vi "Generic - DI1.vi"(0 "VISA session":refnum<visa-resource-name>="MW100", 2 "Semiphore":T2, 5 "Channel_Enum":T1=1 items=["4-20_OUT", "Pres_HI1", "Pres_HI2", "Pres_LOW", "Pres_PIN", "HEATER_TOP", "HEATER_BOT", "T_Shell", "FLOWMETER", "WATT_SENSE", "WH_TICK", "Tc_1", "Tc_2", "Tc_3", "Tc_4", "Tc_5", "Tc_6", "Tc_down", "T_Shell_2", "T_Shell_3", "T_Shell_4", "RTD_IN", "RTD_OUT", "RTD_AMB", "INTF_TEMPFLO", "INTF_READY", "INTF_START", "INTF_STOP", "DRM_LOW", "DRM_HIGH", "PWR_MAIN", "VLV_DUMP", "VLV_OUT", "VLV_IN", "WATT_HOURS", "FLOW(SAMPLE)", "GALLONS", "FLOW(GPM)"], 11 "Error In":errorcluster) -> (4 "dup VISA session":refnum<visa-resource-name>, 6 "Value":bool, 15 "error out":errorcluster)   [LabVIEW 2009]
uses:
  ChannelSettings.ctl
panel:
  out "number":dbl
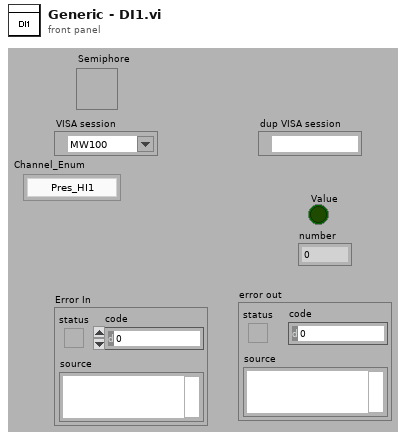
[diagram p1: front panel]
types:
  T1 = typedef "ChannelSettings.ctl" = u32
  T2 = typedef "Semaphore RefNum" = refnum<k1>
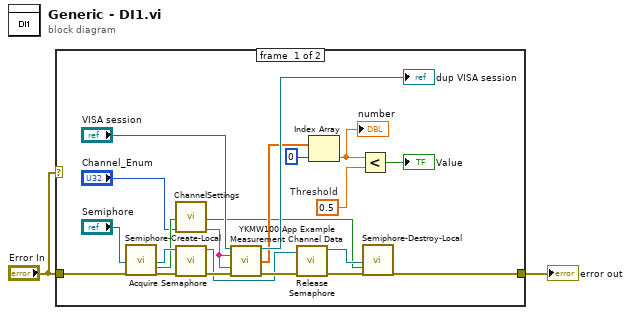
[diagram p0: block diagram]
diagram:
  n1 = case shown="Error" "Error In" {
    tunnel: "Error In" -> [w14 w23]
    tunnel: [w12 w23] -> w2
    frame #0 {
      w17 = 0.5  # Threshold
      n2 = call "Semiphore-Create-Local.vi"("Semiphore"="Semiphore", "error in (no error)"=w14) -> ("semaphore"=w9:T2, "Local?"=w4:bool, "error out"=w11:errorcluster)  [unwired: 15 in]
      n3 = call "ChannelSettings.vi"("Channel_Enum"="Channel_Enum") -> ("Channel String"=w20:string)  [unwired: 10 in]
      n4 = call <vilib>:"Acquire Semaphore.vi"("error in (no error)"=w11, "semaphore"=w9) -> ("error out"=w10:errorcluster, "semaphore out"=w6:T2)  [unwired: 3 in, 1 out]
      n5 = call "YKMW100 App Example Measurement Channel Data.vi"("VISA session"="VISA session", "Start Channel (001)"=w20, "End Channel (001)"=w20, "error in (no error)"=w10) -> ("dup VISA session"=→"dup VISA session":refnum<visa-resource-name>, "Data List"=w16:dbl[], "error out"=w7:errorcluster)  [unwired: 4 in, 5 out]
      n6 = call <vilib>:"Release Semaphore.vi"("error in (no error)"=w7, "semaphore"=w6) -> ("error out"=w8:errorcluster, "semaphore out"=w5:T2)  [unwired: 4 in]
      n7 = Index Array(array=w16, index=0) -> (element=w15:dbl)
      "number" <- w15
      n8 = Less?(x=w15, y=w17) -> (x < y?=→"Value":bool)
      n9 = call "Semiphore-Destroy-Local.vi"("Semiphore"=w5, "Local?"=w4, "error in (no error)"=w8) -> ("error out"=w12:errorcluster)  [unwired: 16 in]
    }
    frame #1 {
    }
  }
  "error out" <- w2
